vi "readTDMS.vi"() -> ()   [LabVIEW 2012]
panel:
  in  "Path":path
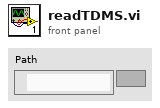
[diagram p1: front panel]
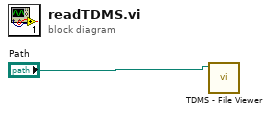
[diagram p0: block diagram]
diagram:
  n1 = call <vilib>:"TDMS - File Viewer.vi"("file path"="Path") -> ()  [unwired: 5 in, 2 out]
